vi "Close.vi"(8 "error in":errorcluster, 11 "DB-SQLite in":refnum<class "DB-SQLite.lvclass">) -> (0 "error out":errorcluster, 3 "DB-SQLite out":refnum<class "DB-SQLite.lvclass">)   [LabVIEW 2020, in "hse-db-sqlite.lvlib" / "DB-SQLite.lvclass"]
doc: "____\nHAMPEL SOFTWARE ENGINEERING v1.4.0 (2023-12-19 09:52)"
uses:
  DB-SQLite.lvclass
  <vilib>/drjdpowell/SQLite Library/SQL Connection/Connection.lvclass
  DB-SQLite.lvclass/DB-SQLite.ctl
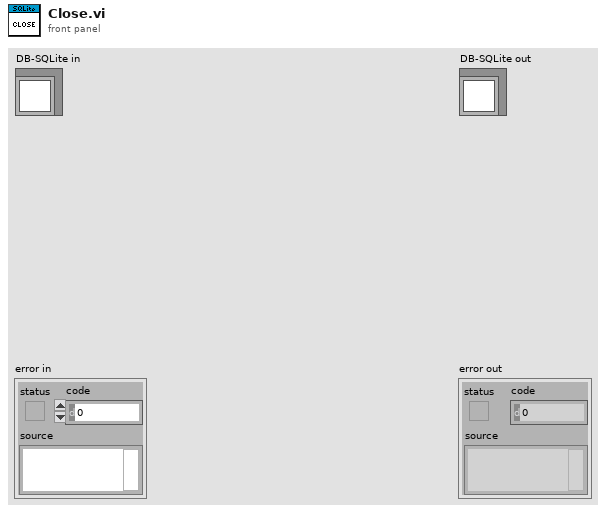
[diagram p1: front panel]
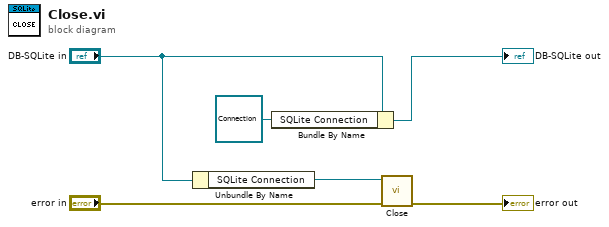
[diagram p0: block diagram]
diagram:
  n1 = Unbundle By Name("DB-SQLite in") -> ("SQLite Connection"=w2:refnum<class "Connection.lvclass">)
  n2 = Bundle By Name(cluster="DB-SQLite in", "SQLite Connection"=refnum<class "Connection.lvclass"> refnum) -> (→"DB-SQLite out":refnum<class "DB-SQLite.lvclass">)
  n3 = call-dynamic "Close.vi"("error in (no error)"="error in", "SQLite Connection in"=w2) -> ("error out"=→"error out":errorcluster)  [unwired: 9 in]
